vi "find best period.vi"(5 "Array of Ch2 desired times":dbl[unit][](array[numeric]), 6 "Array of Ch1 desired times":dbl[unit][](array[numeric])) -> (0 "Array of Ch2 \"period-units\"":i32[](array[numeric]), 1 "Array of Ch2 actual times":dbl[unit][](array[numeric]), 2 "Array of Ch1 \"period-units\"":i32[](array[numeric]), 3 "Array of Ch1 actual times":dbl[unit][](array[numeric]), 4 "best period":dbl[unit])   [LabVIEW 2009]
doc: "This will find the best period (defined as the one with the minimum squared error), given an array of times from channel 1 and an array of times from channel 2."
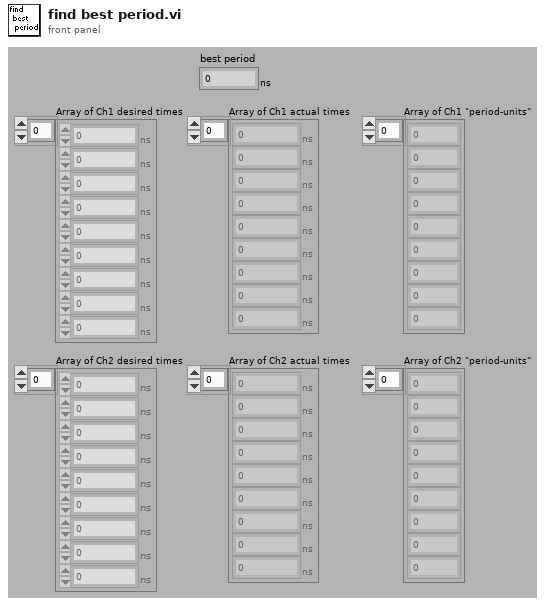
[diagram p1: front panel]
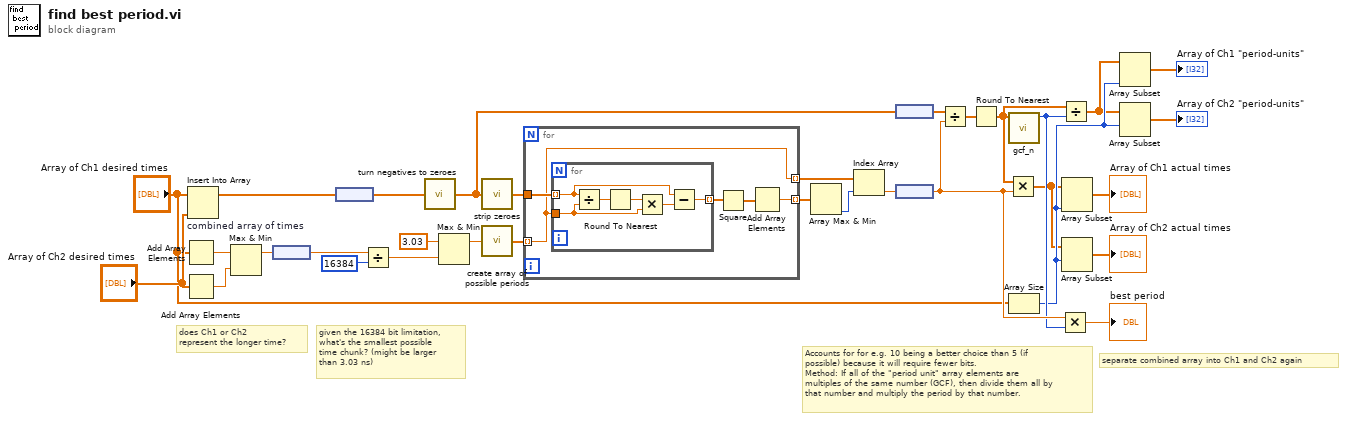
[diagram p0: block diagram]
diagram:
  # "separate combined array into Ch1 and Ch2 again"
  # "Accounts for for e.g. 10 being a better choice than 5 (if\npossible) because it will require fewer bits. \nMethod: If all of the \"period unit\" array elements are\nmultiples of the same number (GCF), then divide them all by\nthat number and multiply the period by that number."
  # "given the 16384 bit limitation, \nwhat's the smallest possible \ntime chunk? (might be larger\nthan 3.03 ns)"
  # "does Ch1 or Ch2 \nrepresent the longer time?"
  n1 = Add Array Elements(numeric array="Array of Ch1 desired times") -> (sum=w24:dbl[unit])
  n2 = Add Array Elements(numeric array="Array of Ch2 desired times") -> (sum=w25:dbl[unit])
  n3 = Insert Into Array "combined array of times"(array="Array of Ch1 desired times", new element="Array of Ch2 desired times") -> (w9:dbl[unit][])  [unwired: 1 in]
  n4 = Max & Min(x=w24, y=w25) -> (max(x,y)=w26:dbl[unit])  [unwired: 1 out]
  n5 = node(w26) -> (w27:dbl)
  n6 = node(w9) -> (w11:dbl[])
  n7 = Divide(x=w27, y=16384) -> (x/y=w32:dbl)
  n8 = call "turn negatives to zeroes.vi"("Array in"=w11) -> ("Array out"=w17:dbl[])
  n9 = Max & Min(x=3.03, y=w32) -> (max(x,y)=w30:dbl)  [unwired: 1 out]
  n10 = call "strip zeroes.vi"("Array in"=w17) -> ("Array out"=w18:dbl[])
  n11 = call "create array of possible periods.vi"("starting number"=w30) -> ("array of possible periods"=w31:dbl[])
  n12 = for {
    tunnel: w18 -> [w37]
    tunnel: [w34] -> w22 mode=indexing
    tunnel: [w36] -> w20 mode=indexing
    tunnel: w31 -> [w36] mode=indexing
    n13 = for {
      tunnel: w37 -> [w40] mode=indexing
      tunnel: w36 -> [w41]
      tunnel: [w38] -> w33 mode=indexing
      n14 = Divide(x=w40, y=w41) -> (x/y=w43:dbl)
      n15 = Round To Nearest(number=w43) -> (nearest integer value=w42:dbl)
      n16 = Multiply(x=w42, y=w41) -> (x*y=w39:dbl)
      n17 = Subtract(x=w40, y=w39) -> (x-y=w38:dbl)
    }
    n18 = Square(x=w33) -> (x^2=w35:dbl[])
    n19 = Add Array Elements(numeric array=w35) -> (sum=w34:dbl)
  }
  n20 = Array Max & Min(array=w22) -> (min index (indices)=w21:i32)  [unwired: 3 out]
  n21 = Index Array(array=w20, index=w21) -> (element=w23:dbl)
  n22 = node(w17) -> (w16:dbl[unit][])
  n23 = node(w23) -> (w14:dbl[unit])
  n24 = Divide(x=w16, y=w14) -> (x/y=w19:dbl[])
  n25 = Round To Nearest(number=w19) -> (nearest integer value=w15:dbl[])
  n26 = Multiply(x=w15, y=w14) -> (x*y=w4:dbl[unit][])
  n27 = call "gcf_n.vi"("Values"=w15) -> ("GCF"=w13:i32)  [unwired: 1 in, 9 out]
  n28 = Array Size(array="Array of Ch1 desired times") -> (size(s)=w5:i32)
  n29 = Multiply(x=w14, y=w13) -> (x*y=→"best period":dbl[unit])
  n30 = Divide(x=w15, y=w13) -> (x/y=w3:dbl[])
  n31 = Array Subset(array=w4, length=w5) -> (→"Array of Ch1 actual times":dbl[unit][])  [unwired: 1 in]
  n32 = Array Subset(array=w4, index=w5) -> (→"Array of Ch2 actual times":dbl[unit][])  [unwired: 1 in]
  n33 = Array Subset(array=w3, length=w5) -> (→"Array of Ch1 \"period-units\"":dbl[])  [unwired: 1 in]
  n34 = Array Subset(array=w3, index=w5) -> (→"Array of Ch2 \"period-units\"":dbl[])  [unwired: 1 in]
